vi "Read.vi"(8 "error in":errorcluster, 11 "Chiller Cluster - 2 Channel.lvclass":refnum<class "Climate Chamber - 2 Channel.lvclass">) -> (0 "error out":errorcluster, 3 "output cluster":refnum<class "Climate Chamber - 2 Channel.lvclass">)   [LabVIEW 2023, in "Climate Chamber - 2 Channel.lvclass"]
uses:
  Climate Chamber - 2 Channel.lvclass
  Climate Chamber - 2 Channel.lvclass/Climate Chamber - 2 Channel.ctl
  4448cff9-e18d-4a6b-945e-10b1e3fd2828.vi
  4a46be96-aeb5-43b7-9243-adca9a8444cf.vi
  27230f32-3038-432e-846c-8983fd03581f.vi
  4448cff9-e18d-4a6b-945e-10b1e3fd2828.vi/c28b0ead-42ad-4072-80a2-aca7f2bd7ce3.vi
  4448cff9-e18d-4a6b-945e-10b1e3fd2828.vi/219d0231-d98b-4193-b5cc-84f90e3c9091.vi
  4a46be96-aeb5-43b7-9243-adca9a8444cf.vi/c28b0ead-42ad-4072-80a2-aca7f2bd7ce3.vi
  4a46be96-aeb5-43b7-9243-adca9a8444cf.vi/219d0231-d98b-4193-b5cc-84f90e3c9091.vi
  27230f32-3038-432e-846c-8983fd03581f.vi/c28b0ead-42ad-4072-80a2-aca7f2bd7ce3.vi
  27230f32-3038-432e-846c-8983fd03581f.vi/219d0231-d98b-4193-b5cc-84f90e3c9091.vi
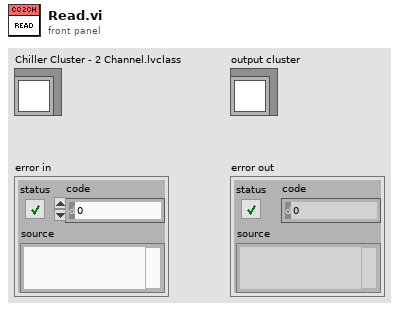
[diagram p1: front panel]
types:
  T1 = cluster{"OnOff.ACT":bool, "ErrorAcknowledge.ACT":bool}
  T2 = cluster{"Temperature.ch01.SP":dbl, "TemperatureMIN.ch01.SP":dbl, "TemperatureMAX.ch01.SP":dbl, "TemperatureGrad.ch01.SP":dbl, "Humidity.ch01.SP":dbl, "HumidityMIN.ch01.SP":dbl, "HumidityMAX.ch01.SP":dbl, "HumidityGrad.ch01.SP":dbl}
  T3 = cluster{"Temperature.ch02.SP":dbl, "TemperatureMIN.ch02.SP":dbl, "TemperatureMAX.ch02.SP":dbl, "TemperatureGrad.ch02.SP":dbl, "Humidity.ch02.SP":dbl, "HumidityMIN.ch02.SP":dbl, "HumidityMAX.ch02.SP":dbl, "HumidityGrad.ch02.SP":dbl}
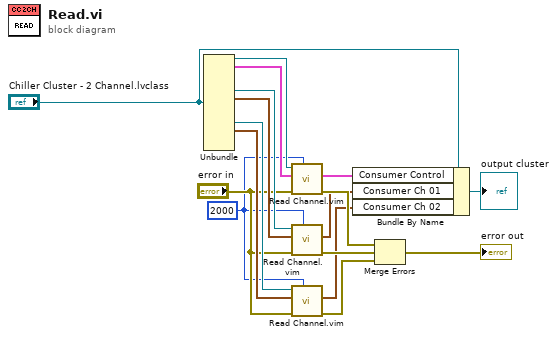
[diagram p0: block diagram]
diagram:
  w3 = 2000 ("Timeout (ms)")
  n1 = Unbundle("Chiller Cluster - 2 Channel.lvclass") -> (w16:refnum<k21>, w15:T1, w8:refnum<k21>, w7:T2, w6:refnum<k21>, w5:T3)  [unwired: 6 out]
  n2 = call "Read Channel.vim"("Timeout (ms)"=w3, "error in"="error in", "Data in"=w15, "ADAS HIL Channel in"=w16) -> ("error out"=w14:errorcluster, "Data out"=w17:T1)  [unwired: 4 in, 2 out]
  n3 = call "Read Channel.vim"("Timeout (ms)"=w3, "error in"="error in", "Data in"=w7, "ADAS HIL Channel in"=w8) -> ("error out"=w13:errorcluster, "Data out"=w9:T2)  [unwired: 4 in, 2 out]
  n4 = call "Read Channel.vim"("Timeout (ms)"=w3, "error in"="error in", "Data in"=w5, "ADAS HIL Channel in"=w6) -> ("error out"=w2:errorcluster, "Data out"=w1:T3)  [unwired: 4 in, 2 out]
  n5 = Bundle By Name(cluster="Chiller Cluster - 2 Channel.lvclass", "Consumer Control"=w17, "Consumer Ch 01"=w9, "Consumer Ch 02"=w1) -> (→"output cluster":refnum<class "Climate Chamber - 2 Channel.lvclass">)
  n6 = Merge Errors(w14, w13, w2) -> (→"error out":errorcluster)
